vi "tcpread.vi"(2 "String 2":string, 3 "TCP Network Connection Refnum":refnum<k5>) -> (0 "OUT":dbl, 1 "TCP Network Connection Refnum 2":refnum<k5>)   [LabVIEW 2014]
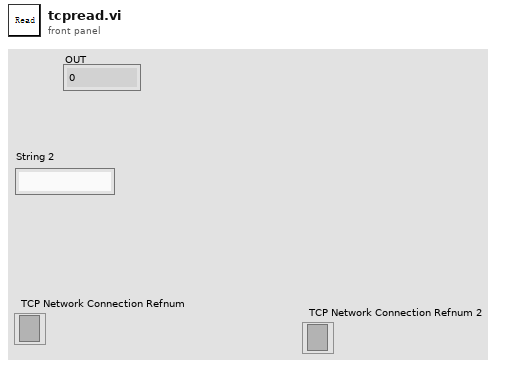
[diagram p1: front panel]
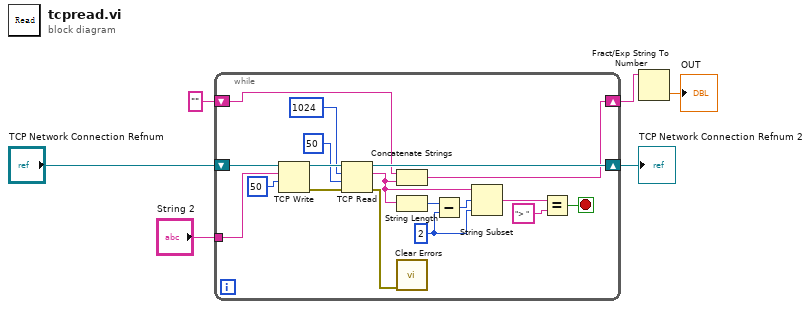
[diagram p0: block diagram]
diagram:
  n1 = while {
    tunnel: "String 2" -> [w20]
    shift-right: [w18] -> w2
    shift-left: "TCP Network Connection Refnum" -> [w19]
    shift-right: [w8] -> w5
    shift-left: "" -> [w10]
    stop <- w14 stop-if-true
    w11 = 2 ("y")
    n2 = TCP Write(connection ID=w19, data in=w20, 9:50 ("timeout ms (25000)")) -> (connection ID out=w23:refnum<k5>, error out=w7:errorcluster)  [unwired: 1 in, 1 out]
    n3 = TCP Read(connection ID=w23, bytes to read=1024, error in (no error)=w7, 9:50 ("timeout ms (25000)")) -> (connection ID out=w18:refnum<k5>, data out=w9:string, error out=w17:errorcluster)  [unwired: 1 in]
    n4 = Concatenate Strings(w10, w9) -> (w8:string)
    n5 = String Length(string=w9) -> (length=w13:i32)
    n6 = call <vilib>:"Clear Errors.vi"("error in (no error)"=w17) -> ()  [unwired: 5 in, 2 out]
    n7 = Subtract(x=w13, y=w11) -> (x-y=w12:i32)
    n8 = String Subset(string=w9, offset (0)=w12, length (rest)=w11) -> (substring=w15:string)
    n9 = Equal?(x=w15, y="> ") -> (x = y?=w14:bool)
  }
  "TCP Network Connection Refnum 2" <- w2
  n10 = Fract/Exp String To Number(string=w5) -> (number=→"OUT":dbl)  [unwired: 3 in, 1 out]
